vi "testStrLength.vi"() -> ()   [LabVIEW 2017]
panel:
  out "Test String Len":i32
  in  "Test String Len 2":string
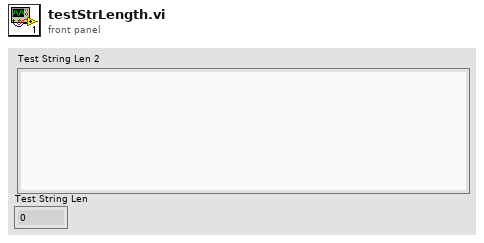
[diagram p1: front panel]
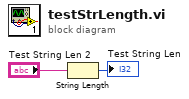
[diagram p0: block diagram]
diagram:
  n1 = String Length(string="Test String Len 2") -> (length=→"Test String Len":i32)
